vi "TF+NLH_2Dsweep.vi"() -> ()   [LabVIEW 2022 SP3]
uses:
  <vilib>/Analysis/baseanly.llb/Mean (DBL).vi
  <vilib>/Utility/file.llb/Write Delimited Spreadsheet (DBL).vi
  <vilib>/Analysis/NI_AALBase.lvlib
panel:
  in  "T Delay":dbl=3600.0
  out "Temperature":dbl
  out "Field":dbl
  out "Field Status 2":i32(ring) items=["MagnetUnknown"=0, "StablePersistent"=1, "WarmingSwitch"=2, "CoolingSwitch"=3, "StableDriven"=4, "Iterating"=5, "Charging"=6, "Discharging"=7, "CurrentError"=8, "MagnetFailure"=15]
  out "Temperature Status 2":i32(ring) items=["TemperatureUnknown"=0, "Stable"=1, "Tracking"=2, "Near"=5, "Chasing"=6, "Filling"=7, "Standby"=10, "Disabled"=13, "ImpedanceNotFunction"=14, "TempFailure"=15]
  in  "?":bool
  out "Sine voltage F":dbl format="%#_13g"
  out "Sine voltage T":dbl format="%#_13g"
  in  "Initialize after measurement":bool
  in  "F Delay":dbl=5.0
  out "PhaseA-F":cluster{dbl[], dbl[]}(graph)
  out "RA-F":cluster{dbl[], dbl[]}(graph)
  out "Phaseh1-F":cluster{dbl[], dbl[]}(graph)
  out "Rh1B-F":cluster{dbl[], dbl[]}(graph)
  out "phase B 2":dbl
  in  "Phase B 2":u16(ring)=9 items=["X", "Y", "R", "Theta", "Frequency", "Noise", "Xh1", "Yh1", "Rh1", "Theta h1", "Xh2", "Yh2", "Rh2", "Theta h2"]
  out "phase A 2":dbl
  in  "Phase A 2":u16(ring)=3 items=["X", "Y", "R", "Theta", "Frequency", "Noise", "Xh1", "Yh1", "Rh1", "Theta h1", "Xh2", "Yh2", "Rh2", "Theta h2"]
  out "para1 Measurement (mV) 2":dbl=1.49013e-07
  in  "F Clear Plot A":bool
  in  "Parameter A 2":u16(ring)=2 items=["X", "Y", "R", "Theta", "Frequency", "Noise", "Xh1", "Yh1", "Rh1", "Theta h1", "Xh2", "Yh2", "Rh2", "Theta h2"]
  out "para2 Measurement (uV) 2":dbl=1.49013e-07
  in  "F Clear Plot B":bool
  in  "Parameter B 2":u16(ring)=8 items=["X", "Y", "R", "Theta", "Frequency", "Noise", "Xh1", "Yh1", "Rh1", "Theta h1", "Xh2", "Yh2", "Rh2", "Theta h2"]
  out "V Loop Run F":i32
  out "Backward":bool
  out "Forward":bool
  in  "V Step(mV)":i32=20
  out "V Loop Run T":i32
  in  "V Loop#":i32=1
  in  "High Value (V)":dbl=3.0
  in  "Low Value (V)":dbl=0.1
  in  "Series Resistance":string="20kOhm"
  in  "System Stablization (s)":dbl=0.1 format="%#_13g"
  in  "Low Value (Oe)":dbl
  in  "High Value (Oe)":dbl=70000.0
  in  "Sweep Field Approach":i32(ring) items=["Linear", "NoOvershoot", "Oscillate"]
  in  "Sweep F Rate (Oe/s)":dbl=200.0 format="%#_13g"
  in  "Sweep F mode":i32(ring) items=["Persistent", "Driven"]
  in  "Set Fixed T":dbl=300.0
  in  "Fixed Temperature Approach":i32(ring)=1 items=["FastSettle", "NoOvershoot"]
  in  "FIxed T  Rate (K/min)":dbl=20.0
  out "Field Setting":dbl format="%#_13g"
  out "Fixed Temperature":dbl
  out "Measured Field":dbl
  out "Field Status":i32(ring) items=["MagnetUnknown"=0, "StablePersistent"=1, "WarmingSwitch"=2, "CoolingSwitch"=3, "StableDriven"=4, "Iterating"=5, "Charging"=6, "Discharging"=7, "CurrentError"=8, "MagnetFailure"=15]
  out "Temperature Status":i32(ring) items=["TemperatureUnknown"=0, "Stable"=1, "Tracking"=2, "Near"=5, "Chasing"=6, "Filling"=7, "Standby"=10, "Disabled"=13, "ImpedanceNotFunction"=14, "TempFailure"=15]
  out "Measuring F":bool
  in  "Step(Oe)":i32=5000
  out "Temperature Status":i32(ring) items=["TemperatureUnknown"=0, "Stable"=1, "Tracking"=2, "Near"=5, "Chasing"=6, "Filling"=7, "Standby"=10, "Disabled"=13, "ImpedanceNotFunction"=14, "TempFailure"=15]
  out "Field Status":i32(ring) items=["MagnetUnknown"=0, "StablePersistent"=1, "WarmingSwitch"=2, "CoolingSwitch"=3, "StableDriven"=4, "Iterating"=5, "Charging"=6, "Discharging"=7, "CurrentError"=8, "MagnetFailure"=15]
  out "Fixed Field":dbl
  out "Measured Temperature":dbl
  in  "Set FIxed F (Oe)":dbl format="%#_13g"
  in  "Fixed Field Approach":i32(ring) items=["Linear", "NoOvershoot", "Oscillate"]
  in  "FIxed F Rate (Oe/s)":dbl=100.0 format="%#_13g"
  in  "Fixed F mode":i32(ring) items=["Persistent", "Driven"]
  in  "Sweep Temperature Approach":i32(ring)=1 items=["FastSettle", "NoOvershoot"]
  in  "Sweep T  Rate (K/min)":dbl=10.0
  in  "Sweep T/F":bool=TRUE
  in  "Remote":bool=TRUE
  in  "IP Address":string="169.254.170.239"
  out "Measuring T":bool
  in  "path (folder + filename)":string="G:\\My Drive\\Opticool\\Measurement\\NLH\\T dependence\\TaI23_A67_B68_267Hz"
  in  "LOCKIN address":refnum<visa-resource-name>="COM3"
  out "PhaseA-T":cluster{dbl[], dbl[]}(graph)
  out "RA-T":cluster{dbl[], dbl[]}(graph)
  out "Phaseh1-T":cluster{dbl[], dbl[]}(graph)
  out "Rh1B-T":cluster{dbl[], dbl[]}(graph)
  out "phase B":dbl
  in  "Phase B":u16(ring)=9 items=["X", "Y", "R", "Theta", "Frequency", "Noise", "Xh1", "Yh1", "Rh1", "Theta h1", "Xh2", "Yh2", "Rh2", "Theta h2"]
  out "phase A":dbl
  in  "Phase A":u16(ring)=3 items=["X", "Y", "R", "Theta", "Frequency", "Noise", "Xh1", "Yh1", "Rh1", "Theta h1", "Xh2", "Yh2", "Rh2", "Theta h2"]
  out "para1 Measurement (mV)":dbl=1.49013e-07
  in  "T Clear Plot A":bool
  in  "Parameter A":u16(ring)=2 items=["X", "Y", "R", "Theta", "Frequency", "Noise", "Xh1", "Yh1", "Rh1", "Theta h1", "Xh2", "Yh2", "Rh2", "Theta h2"]
  out "para2 Measurement (uV)":dbl=1.49013e-07
  in  "T Clear Plot B":bool
  in  "Parameter B":u16(ring)=8 items=["X", "Y", "R", "Theta", "Frequency", "Noise", "Xh1", "Yh1", "Rh1", "Theta h1", "Xh2", "Yh2", "Rh2", "Theta h2"]
  out "Temperature Setting":dbl format="%#_13g"
  in  "Save data or not":bool=TRUE
  in  "Step(K)":i32=10
  in  "B frequency":dbl=267.77 format="%#_13g"
  in  "B Input Connection (0: Single-Ended)":u16(ring)=1 items=["Single-Ended Voltage", "Differential Voltage", "1 MOhm Current Gain", "100 MOhm Current Gain"]
  in  "B harmonic 1":u8=2
  in  "B harmonic 2":u8=3
  in  "B reference Manual Phase":dbl=90.0
  in  "auto phase B":bool=TRUE
  in  "B Sample time (s)":dbl=0.001 min=0.001 max=100.0 step=0.001
  in  "B Sensitivity":u16(ring)=21 items=["1 nV/fA", "2 nV/fA", "5 nV/fA", "10 nV/fA", "20 nV/fA", "50 nV/fA", "100 nV/fA", "200 nV/fA", "500 nV/fA", "1 uV/pA", "2 uV/pA", "5 uV/pA", "10 uV/pA", "20 uV/pA", "50 uV/pA", "100 uV/pA", "200 uV/pA", "500 uV/pA", "1 mV/nA", "2 mV/nA", "5 mV/nA", "10 mV/nA", "20 mV/nA", "50 mV/nA", "100 mV/nA", "200 mV/nA", "500 mV/nA", "1 V/uA"]
  in  "Enable Sync Filter B (open when f<200Hz)":bool
  in  "B Time Constant":u8(ring)=9 items=["10 us", "30 us", "100 us", "300 us", "1 ms", "3 ms", "10 ms", "30 ms", "100 ms", "300 ms", "1 s", "3 s", "10 s", "30 s", "100 s", "300 s", "1 ks", "3 ks"]
  in  "B Reference Source":u8(ring) items=["External", "Internal", "Internal Sweep", "Channel-A"]
  in  "B Low Pass Filter Slope":u8(ring)=2 items=["6 dB/oct", "12 dB/oct", "18 db/oct", "24 dB/oct"]
  in  "A frequency":dbl=267.77 format="%#_13g"
  in  "A Input Connection (0: Single-Ended)":u16(ring)=1 items=["Single-Ended Voltage", "Differential Voltage", "1 MOhm Current Gain", "100 MOhm Current Gain"]
  in  "A harmonic 1":u8=2
  in  "A harmonic 2":u8=3
  in  "A reference Manual Phase":dbl
  in  "auto phase A":bool=TRUE
  in  "A Reference Source":u8(ring)=1 items=["External", "Internal", "Internal Sweep"]
  in  "A Sample time (s)":dbl=0.001 min=0.001 max=100.0 step=0.001
  in  "A Time Constant":u8(ring)=8 items=["10 us", "30 us", "100 us", "300 us", "1 ms", "3 ms", "10 ms", "30 ms", "100 ms", "300 ms", "1 s", "3 s", "10 s", "30 s", "100 s", "300 s", "1 ks", "3 ks"]
  in  "Enable Sync Filter A (open when f<200Hz)":bool
  in  "A Sensitivity":u16(ring)=21 items=["1 nV/fA", "2 nV/fA", "5 nV/fA", "10 nV/fA", "20 nV/fA", "50 nV/fA", "100 nV/fA", "200 nV/fA", "500 nV/fA", "1 uV/pA", "2 uV/pA", "5 uV/pA", "10 uV/pA", "20 uV/pA", "50 uV/pA", "100 uV/pA", "200 uV/pA", "500 uV/pA", "1 mV/nA", "2 mV/nA", "5 mV/nA", "10 mV/nA", "20 mV/nA", "50 mV/nA", "100 mV/nA", "200 mV/nA", "500 mV/nA", "1 V/uA"]
  in  "A Low Pass Filter Slope":u8(ring)=2 items=["6 dB/oct", "12 dB/oct", "18 db/oct", "24 dB/oct"]
  in  "stabilization(S)":dbl=0.1 format="%#_13g"
  in  "End Value (K)":dbl=302.0
  in  "Start Value (K)":dbl=2.0
  in  "Single/Double":i32=2 min=1 max=2 step=1
  # "Statue"
  # "Lock-in Setting"
  # "Channel B"
  # "Channel A"
  # "Sweep Setting"
  # "Sweep F Mesurement"
  # "Temprature and Field Setting"
  # "Sweep T Mesurement"
  # "Sweep F"
  # "Sweep T"
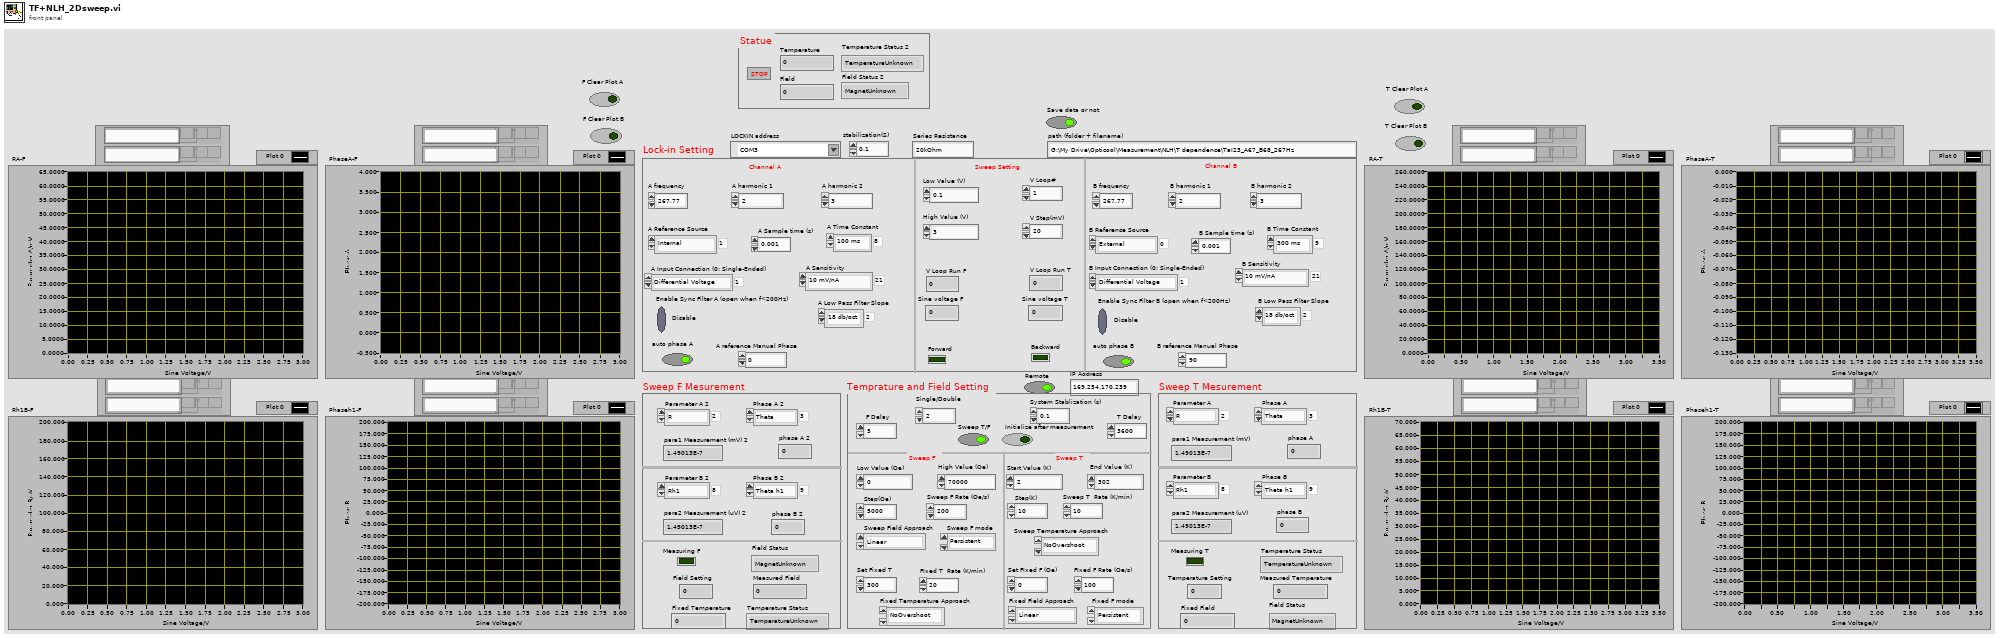
[diagram p1: front panel]
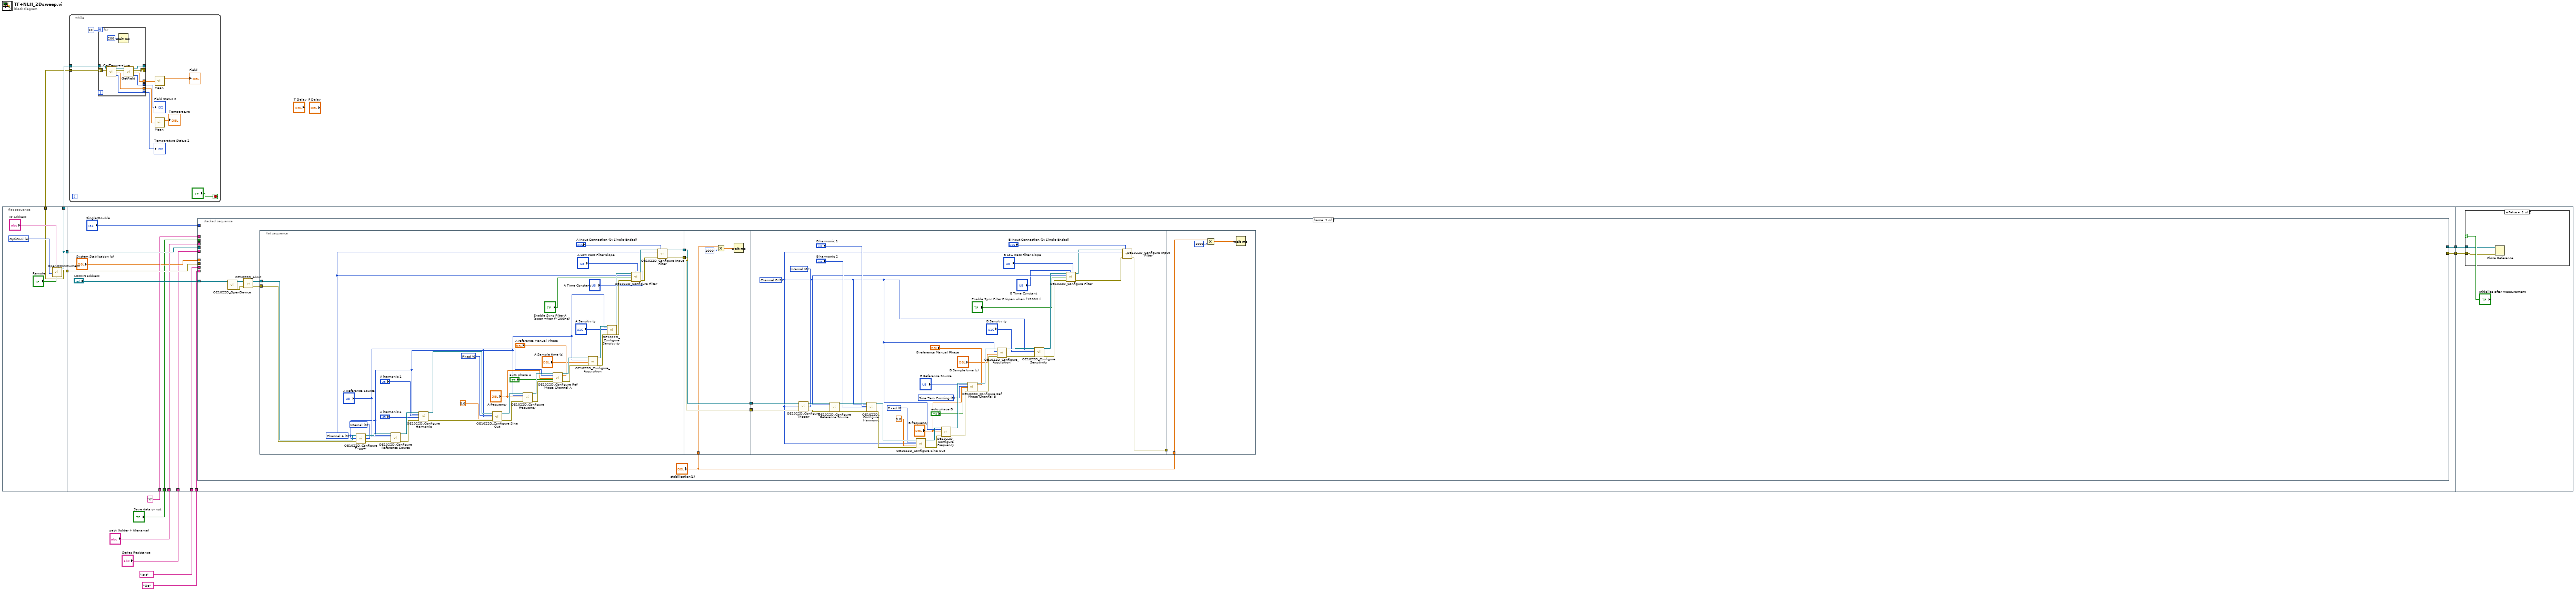
[diagram p0: block diagram]
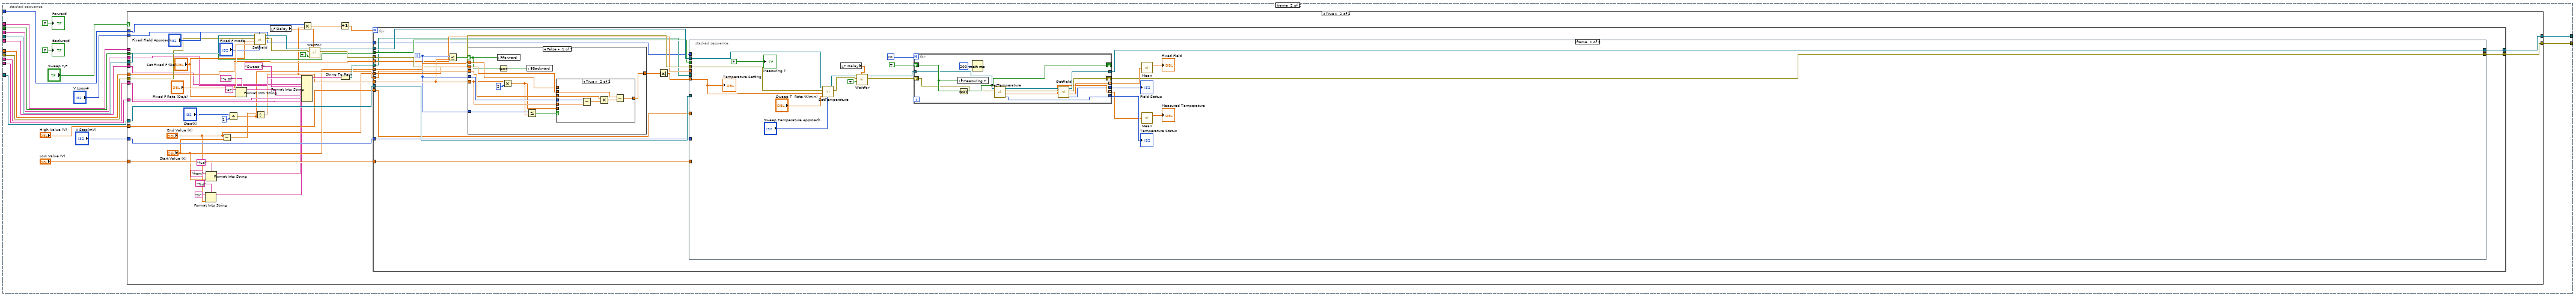
[diagram p2: hidden frame]
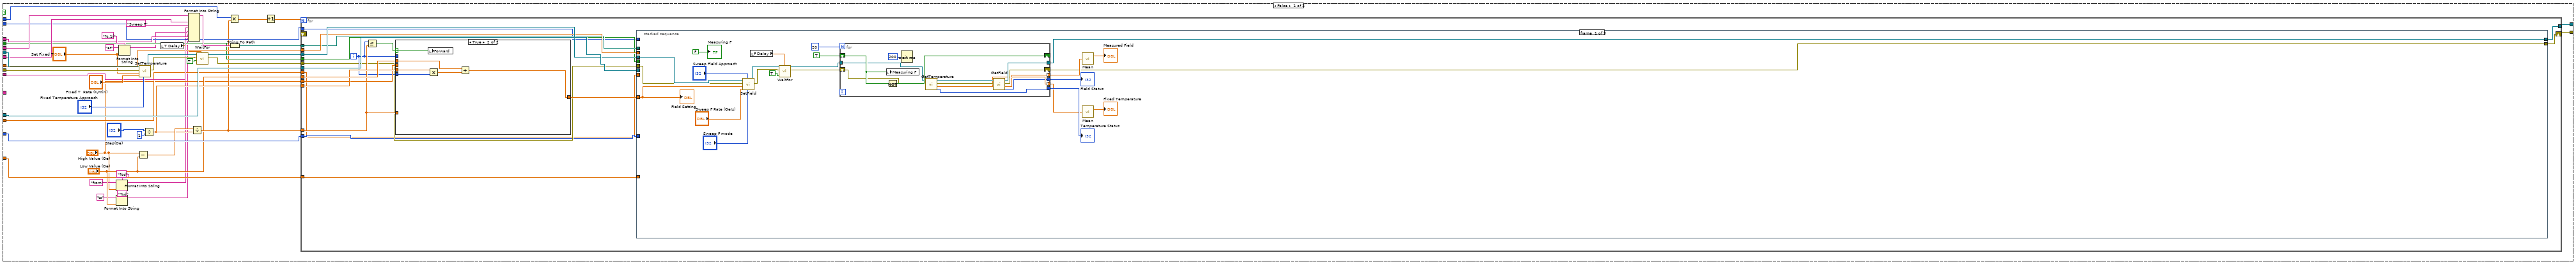
[diagram p3: hidden frame]
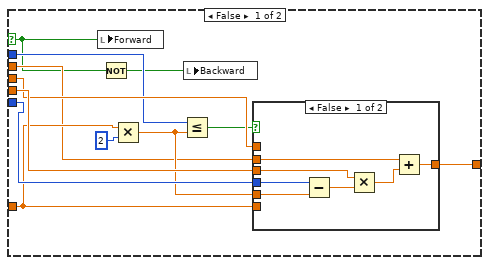
[diagram p4: hidden frame]
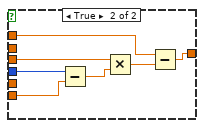
[diagram p5: hidden frame]
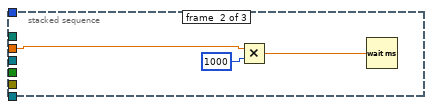
[diagram p6: hidden frame]
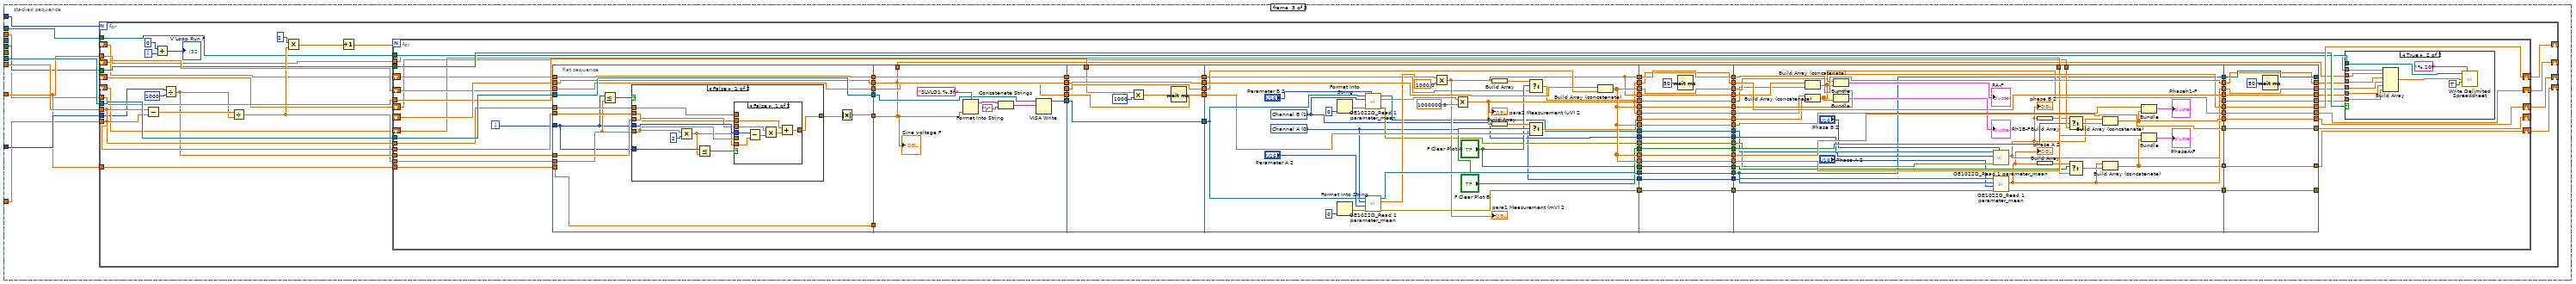
[diagram p7: hidden frame]
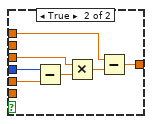
[diagram p9: hidden frame]
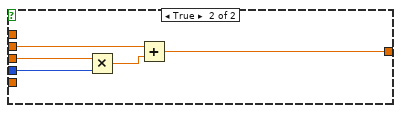
[diagram p10: hidden frame]
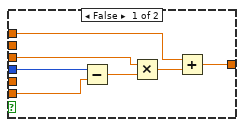
[diagram p11: hidden frame]
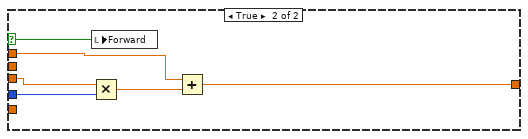
[diagram p12: hidden frame]
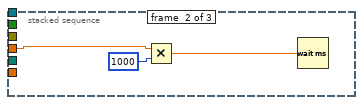
[diagram p13: hidden frame]
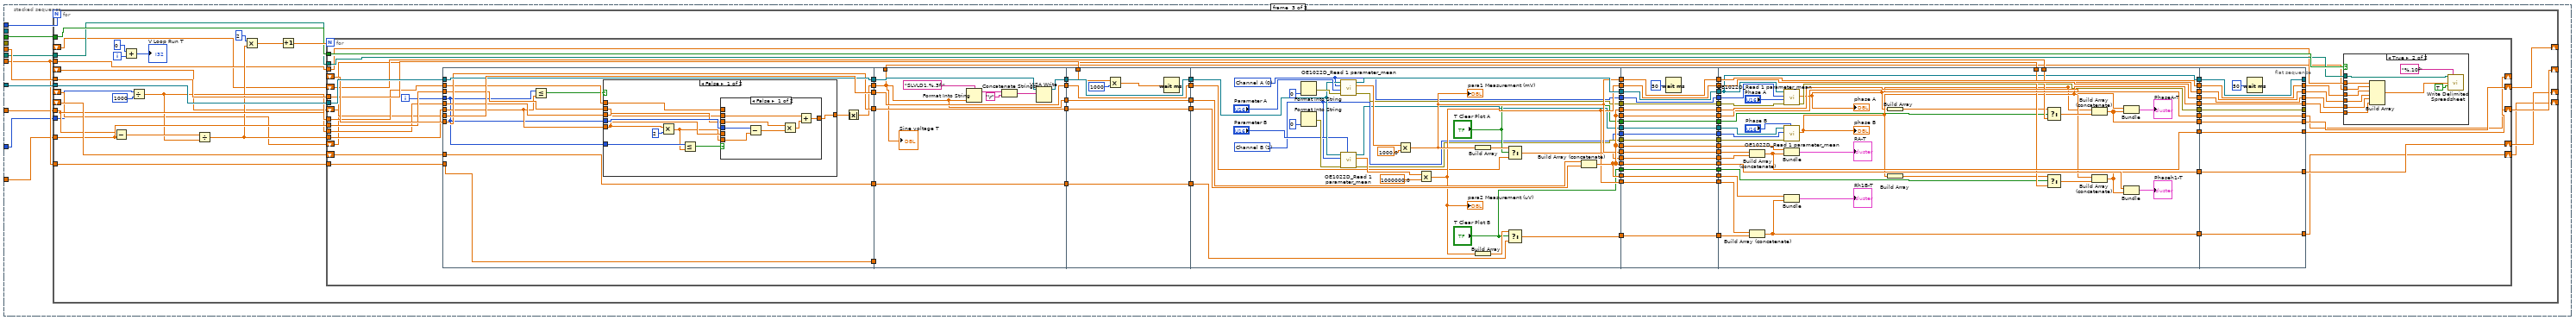
[diagram p14: hidden frame]
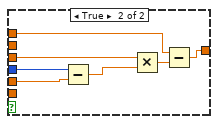
[diagram p16: hidden frame]
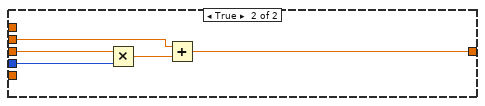
[diagram p17: hidden frame]
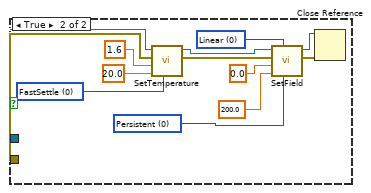
[diagram p18: hidden frame]
diagram:
  n1 = flat-sequence {
    tunnel: [w14] -> w12
    tunnel: [w13] -> w11
    tunnel: [w14] -> w2
    tunnel: [w13] -> w1
    tunnel: w12 -> [w28]
    tunnel: w11 -> [w27]
    tunnel: "path (folder + filename)" -> [w26]
    tunnel: "Oe" -> [w25]
    tunnel: "K" -> [w24]
    tunnel: ".txt" -> [w23]
    tunnel: [w21] -> w6
    tunnel: [w20] -> w5
    tunnel: "Series Resistance" -> [w19]
    tunnel: "Save data or not" -> [w18]
    tunnel: w6 -> [w1015]
    tunnel: w5 -> [w1014]
    frame #0 {
      w15 = 4 items=["PPMS", "VersaLab", "DynaCool", "SVSM", "OptiCool"] ("InstrumentType")
      n2 = call "OpenQDInstrument.vi"("Remote"="Remote", "IP Address"="IP Address", "InstrumentType"=w15) -> ("error out"=w13:errorcluster, "Instrument Ref"=w14:refnum<k24>)  [unwired: 5 in]
    }
    frame #1 {
      n3 = stacked-sequence {
        tunnel: "LOCKIN address" -> [w33 w145]
        tunnel: "Single/Double" -> [_ w144]
        tunnel: w28 -> [_ w142]
        tunnel: w27 -> [_ w141]
        tunnel: w26 -> [_ w140]
        tunnel: w25 -> [_ w139]
        tunnel: w24 -> [_ w138]
        tunnel: w23 -> [_ w137]
        tunnel: "System Stablization (s)" -> [_ w136]
        tunnel: [_ w135] -> w21
        tunnel: [_ w134] -> w20
        tunnel: w19 -> [_ w133]
        tunnel: w18 -> [_ w132]
        frame #0 {
          n4 = call <instrlib>:"OE1022D_OpenDevice.vi"("VISA resource name"=w33) -> ("VISA资源名称输出"=w32:refnum<visa-resource-name>, "错误输出"=w34:errorcluster)  [unwired: 17 in]
          n5 = call <instrlib>:"OE1022D_Abort.vi"("error in (no error)"=w34, "VISA resource name"=w32) -> ("error out"=w39:errorcluster, "VISA resource name out"=w40:refnum<visa-resource-name>)
          n6 = flat-sequence {
            tunnel: w40 -> [w79]
            tunnel: [w67] -> w38
            tunnel: w39 -> [w78]
            tunnel: [w55] -> w36
            tunnel: w38 -> [w84]
            tunnel: [w84] -> w37
            tunnel: w36 -> [w83]
            tunnel: [w83] -> w35
            tunnel: "stabilization(S)" -> [w80]
            tunnel: w37 -> [w105]
            tunnel: [w104] -> w41
            tunnel: w35 -> [w103]
            tunnel: w41 -> [_]
            tunnel: "stabilization(S)" -> [w123]
            frame #0 {
              w54 = u8 0 items=["Fixed", "Linear", "Log"] ("SineOut Mode")
              w56 = u16 0 items=["Internal", "External"] ("Trigger Source (0: Internal)")
              w45 = u8 0 items=["Channel A", "Channel B"] ("OE1022D A/B")
              n7 = call <instrlib>:"OE1022D_Configure Trigger.vi"("Trigger Source (0: Internal)"=w56, "error in (no error)   2"=w78, "OE1022D A/B"=w45, "VISA resource name   2"=w79) -> ("error out   2"=w72:errorcluster, "VISA resource name out   2"=w73:refnum<visa-resource-name>)
              n8 = call <instrlib>:"OE1022D_Configure Reference Source.vi"("VISA resource name"=w73, "OE1022D A/B"=w45, "Reference Source"="A Reference Source", "error in (no error)"=w72) -> ("VISA resource name out"=w71:refnum<visa-resource-name>, "error out"=w69:errorcluster)  [unwired: 14 in]
              n9 = call <instrlib>:"OE1022D_Configure Harmonic.vi"("VISA resource name"=w71, "OE1022D A/B"=w45, "Harmonic 1"="A harmonic 1", "Harmonic 2"="A harmonic 2", "error in (no error)"=w69) -> ("VISA resource name out"=w70:refnum<visa-resource-name>, "error out"=w68:errorcluster)  [unwired: 13 in]
              n10 = call <instrlib>:"OE1022D_Configure Sine Out.vi"("VISA resource name"=w70, "SineOut Mode"=w54, "OE1022D A/B"=w45, "Sine Output Amplitude (V)"=sgl 0.0 ("A Sine Output Amplitude (V)"), "error in (no error)"=w68) -> ("VISA resource name out"=w76:refnum<visa-resource-name>, "error out"=w75:errorcluster)  [unwired: 9 in]
              n11 = call <instrlib>:"OE1022D_Configure Frequency.vi"("VISA resource name"=w76, "OE1022D A/B"=w45, "Internal Frequency(Hz)"="A frequency", "error in (no error)"=w75) -> ("VISA resource name out"=w66:refnum<visa-resource-name>, "error out"=w63:errorcluster)  [unwired: 14 in]
              n12 = call <instrlib>:"OE1022D_Configure Ref Phase Channel A.vi"("VISA resource name"=w66, "Reference Source"="A Reference Source", "Internal Frequency(Hz)"="A frequency", "Auto Phase (T: Enabled)"="auto phase A", "error in (no error)"=w63, "Manual Phase  (degree)"="A reference Manual Phase") -> ("VISA resource name out"=w65:refnum<visa-resource-name>, "error out"=w64:errorcluster)  [unwired: 12 in]
              n13 = call <instrlib>:"OE1022D_Configure_Acquisition.vi"("VISA resource name"=w65, "OE1022D A/B"=w45, "Sample time (s)"="A Sample time (s)", "error in (no error)"=w64) -> ("VISA resource name out"=w48:refnum<visa-resource-name>, "error out"=w47:errorcluster)  [unwired: 4 in]
              n14 = call <instrlib>:"OE1022D_Configure Sensitivity.vi"("VISA resource name"=w48, "OE1022D A/B"=w45, "Sensitivity"="A Sensitivity", "error in (no error)"=w47) -> ("VISA resource name out"=w52:refnum<visa-resource-name>, "error out"=w51:errorcluster)  [unwired: 14 in]
              n15 = call <instrlib>:"OE1022D_Configure Filter.vi"("Low Pass Filter Slope (1: 12dB/oct)"="A Low Pass Filter Slope", "Time Constant (8: 100ms)"="A Time Constant", "error in (no error)"=w51, "Enable Sync Filter (F: Disable)"="Enable Sync Filter A (open when f<200Hz)", "OE1022D A/B"=w45, "VISA resource name"=w52) -> ("error out"=w49:errorcluster, "VISA resource name out"=w50:refnum<visa-resource-name>)  [unwired: 4 in]
              n16 = call <instrlib>:"OE1022D_Configure Input Filter.vi"("VISA resource name"=w50, "Input Source"="A Input Connection (0: Single-Ended)", "OE1022D A/B"=w45, "error in (no error)"=w49) -> ("VISA resource name out"=w55:refnum<visa-resource-name>, "error out"=w67:errorcluster)  [unwired: 10 in]
            }
            frame #1 {
              n17 = Multiply(x=w80, y=1000) -> (x*y=w82:dbl)
              n18 = Wait (ms)(milliseconds to wait=w82) -> ()  [unwired: 1 out]
            }
            frame #2 {
              w87 = u8 2 items=["TTL Pos", "TTL Neg", "Sine Zero Crossing"] ("External Ref Trigger")
              w100 = u8 0 items=["Fixed", "Linear", "Log"] ("SineOut Mode")
              w106 = u16 0 items=["Internal", "External"] ("Trigger Source (0: Internal)")
              w92 = u8 1 items=["Channel A", "Channel B"] ("OE1022D A/B")
              n19 = call <instrlib>:"OE1022D_Configure Trigger.vi"("Trigger Source (0: Internal)"=w106, "error in (no error)   2"=w105, "OE1022D A/B"=w92, "VISA resource name   2"=w103) -> ("error out   2"=w118:errorcluster, "VISA resource name out   2"=w119:refnum<visa-resource-name>)
              n20 = call <instrlib>:"OE1022D_Configure Reference Source.vi"("VISA resource name"=w119, "OE1022D A/B"=w92, "error in (no error)"=w118) -> ("VISA resource name out"=w117:refnum<visa-resource-name>, "error out"=w115:errorcluster)  [unwired: 15 in]
              n21 = call <instrlib>:"OE1022D_Configure Harmonic.vi"("VISA resource name"=w117, "OE1022D A/B"=w92, "Harmonic 1"="B harmonic 1", "Harmonic 2"="B harmonic 2", "error in (no error)"=w115) -> ("VISA resource name out"=w116:refnum<visa-resource-name>, "error out"=w114:errorcluster)  [unwired: 13 in]
              n22 = call <instrlib>:"OE1022D_Configure Sine Out.vi"("VISA resource name"=w116, "SineOut Mode"=w100, "OE1022D A/B"=w92, "Sine Output Amplitude (V)"=sgl 0.0, "error in (no error)"=w114) -> ("VISA resource name out"=w121:refnum<visa-resource-name>, "error out"=w120:errorcluster)  [unwired: 9 in]
              n23 = call <instrlib>:"OE1022D_Configure Frequency.vi"("VISA resource name"=w121, "OE1022D A/B"=w92, "Internal Frequency(Hz)"="B frequency", "error in (no error)"=w120) -> ("VISA resource name out"=w113:refnum<visa-resource-name>, "error out"=w110:errorcluster)  [unwired: 14 in]
              n24 = call <instrlib>:"OE1022D_Configure Ref Phase Channel B.vi"("VISA resource name"=w113, "Reference Source"="B Reference Source", "External Ref Trigger"=w87, "Internal Frequency(Hz)"="B frequency", "Auto Phase (T: Enabled)"="auto phase B", "error in (no error)"=w110, "Manual Phase  (degree)"="B reference Manual Phase") -> ("VISA resource name out"=w112:refnum<visa-resource-name>, "error out"=w111:errorcluster)  [unwired: 11 in]
              n25 = call <instrlib>:"OE1022D_Configure_Acquisition.vi"("VISA resource name"=w112, "OE1022D A/B"=w92, "Sample time (s)"="B Sample time (s)", "error in (no error)"=w111) -> ("VISA resource name out"=w93:refnum<visa-resource-name>, "error out"=w94:errorcluster)  [unwired: 4 in]
              n26 = call <instrlib>:"OE1022D_Configure Sensitivity.vi"("VISA resource name"=w93, "OE1022D A/B"=w92, "Sensitivity"="B Sensitivity", "error in (no error)"=w94) -> ("VISA resource name out"=w97:refnum<visa-resource-name>, "error out"=w96:errorcluster)  [unwired: 14 in]
              n27 = call <instrlib>:"OE1022D_Configure Filter.vi"("Low Pass Filter Slope (1: 12dB/oct)"="B Low Pass Filter Slope", "Time Constant (8: 100ms)"="B Time Constant", "error in (no error)"=w96, "Enable Sync Filter (F: Disable)"="Enable Sync Filter B (open when f<200Hz)", "OE1022D A/B"=w92, "VISA resource name"=w97) -> ("error out"=w95:errorcluster, "VISA resource name out"=w85:refnum<visa-resource-name>)  [unwired: 4 in]
              n28 = call <instrlib>:"OE1022D_Configure Input Filter.vi"("VISA resource name"=w85, "Input Source"="B Input Connection (0: Single-Ended)", "OE1022D A/B"=w92, "error in (no error)"=w95) -> ("error out"=w104:errorcluster)  [unwired: 10 in, 1 out]
            }
            frame #3 {
              n29 = Multiply(x=w123, y=1000) -> (x*y=w125:dbl)
              n30 = Wait (ms)(milliseconds to wait=w125) -> ()  [unwired: 1 out]
            }
          }
        }
        frame #1 {
          n31 = case shown="True" "Sweep T/F" {
            tunnel: w145 -> [w191 w625]
            tunnel: w144 -> [w157 w624]
            tunnel: w142 -> [w184 w620]
            tunnel: w141 -> [w185 w619]
            tunnel: w140 -> [w177 w609]
            tunnel: w139 -> [_ w601]
            tunnel: w138 -> [w170 _]
            tunnel: w137 -> [w176 w607]
            tunnel: w136 -> [w175 w606]
            tunnel: [w174 w605] -> w135
            tunnel: [w173 w604] -> w134
            tunnel: w133 -> [w172 w603]
            tunnel: w132 -> [w166 w600]
            tunnel: "V Step(mV)" -> [w169 w592]
            tunnel: "High Value (V)" -> [w167 w591]
            tunnel: "Low Value (V)" -> [w168 w590]
            tunnel: "V Loop#" -> [w165 w589]
            frame False {
              n32 = Format Into String(format string="%d", initial string="from", "High Value (Oe)") -> (resulting string=w148:string)  [unwired: 1 in, 1 out]
              n33 = Format Into String(format string="%d", initial string="to", "Low Value (Oe)") -> (resulting string=w147:string)  [unwired: 1 in, 1 out]
              n34 = Format Into String(format string="%.1f", initial string="at", "Set Fixed T") -> (resulting string=w156:string)  [unwired: 1 in, 1 out]
              n35 = Subtract(x="High Value (Oe)", y="Low Value (Oe)") -> (x-y=w162:dbl)
              n36 = call "SetTemperature.vi"("Approach"="Fixed Temperature Approach", "Rate"="FIxed T  Rate (K/min)", "Temperature"="Set Fixed T", "error in (no error)"=w185, "Instrument Ref In"=w184) -> ("error out"=w186:errorcluster, "Instrument Ref Out"=w187:refnum<k24>)  [unwired: 2 in, 1 out]
              n37 = Divide(x="Step(Oe)", y=1) -> (x/y=w161:dbl)
              n38 = local read "T Delay"() -> (w146:dbl)
              n39 = Format Into String(initial string=w177, w172, "Sweep F", w148, w147, w156, w170, w176) -> (resulting string=w179:string)  [unwired: 2 in, 1 out]
              n40 = Divide(x=w162, y=w161) -> (x/y=w160:dbl)
              n41 = call "WaitFor.vi"("Delay"=w146, "Wait For Temperature"=TRUE ("WaitForTemperature"), "error in (no error)"=w186, "Instrument Ref In"=w187) -> ("error out"=w183:errorcluster, "Instrument Ref Out"=w182:refnum<k24>)  [unwired: 6 in]
              n42 = Multiply(x=w157, y=w160) -> (x*y=w159:dbl)
              n43 = String To Path(string=w179) -> (path=w178:path)
              n44 = Increment(x=w159) -> (x+1=w158:dbl)
              n45 = for {
                N: w158 -> [_]
                tunnel: w191 -> [w210]
                tunnel: w161 -> [w207]
                tunnel: w160 -> [w205]
                tunnel: "Low Value (Oe)" -> [w208]
                tunnel: "High Value (Oe)" -> [w206]
                tunnel: w178 -> [w197]
                tunnel: w182 -> [w202]
                tunnel: w183 -> [w201]
                tunnel: w175 -> [w200]
                shift-right: [w199] -> w174
                shift-left: _ -> [_]
                tunnel: [w198] -> w173
                tunnel: w169 -> [w196]
                tunnel: w168 -> [w195]
                tunnel: w167 -> [w194]
                tunnel: w166 -> [w193]
                tunnel: w165 -> [w192]
                i -> [w204]
                n46 = Less Or Equal?(x=w204, y=w205) -> (x <= y?=w209:bool)
                n47 = case shown="True" w209 {
                  selector: w209 -> [w211 w237]
                  tunnel: w208 -> [w213 w242]
                  tunnel: w204 -> [w222 w241]
                  tunnel: w207 -> [w221 w240]
                  tunnel: [w219 w238] -> w203
                  tunnel: w206 -> [w220 _]
                  tunnel: w205 -> [w215 _]
                  tunnel: w204 -> [w218 _]
                  frame False {
                    n48 = local write "Forward"(w211) -> ()
                    n49 = Not(x=w211) -> (.not. x?=w212:bool)
                    n50 = Multiply(x=w215, y=2) -> (x*y=w214:dbl)
                    n51 = Less Or Equal?(x=w218, y=w214) -> (x <= y?=w216:bool)
                    n52 = local write "Backward"(w212) -> ()
                    n53 = case shown="False" w216 {
                      tunnel: w222 -> [w229 w236]
                      tunnel: w221 -> [w227 w234]
                      tunnel: w220 -> [_ w232]
                      tunnel: [w225 w231] -> w219
                      tunnel: w215 -> [_ w230]
                      tunnel: w214 -> [w224 _]
                      tunnel: w213 -> [w223 _]
                      frame False {
                        n54 = Subtract(x=w229, y=w224) -> (x-y=w228:dbl)
                        n55 = Multiply(x=w227, y=w228) -> (x*y=w226:dbl)
                        n56 = Add(x=w223, y=w226) -> (x+y=w225:dbl)
                      }
                      frame True {
                        n57 = Subtract(x=w236, y=w230) -> (x-y=w235:dbl)
                        n58 = Multiply(x=w234, y=w235) -> (x*y=w233:dbl)
                        n59 = Subtract(x=w232, y=w233) -> (x-y=w231:dbl)
                      }
                    }
                  }
                  frame True {
                    n60 = Multiply(x=w240, y=w241) -> (x*y=w239:dbl)
                    n61 = local write "Forward"(w237) -> ()
                    n62 = Add(x=w242, y=w239) -> (x+y=w238:dbl)
                  }
                }
                n63 = stacked-sequence {
                  tunnel: w210 -> [_ _ w286]
                  tunnel: w203 -> [w248 _ w285]
                  tunnel: w202 -> [w247 _ _]
                  tunnel: w201 -> [w246 _ _]
                  tunnel: w200 -> [_ w279 w283]
                  tunnel: [w245 _ _] -> w199
                  tunnel: [w244 _ _] -> w198
                  tunnel: w197 -> [_ _ w290]
                  tunnel: w196 -> [_ _ w289]
                  tunnel: w195 -> [_ _ w288]
                  tunnel: w194 -> [_ _ w287]
                  tunnel: w193 -> [_ _ w284]
                  tunnel: w192 -> [_ _ w282]
                  frame #0 {
                    n64 = call "SetField.vi"("Mode"="Sweep F mode", "Approach"="Sweep Field Approach", "Rate"="Sweep F Rate (Oe/s)", "Field"=w248, "error in (no error)"=w246, "Instrument Ref In"=w247) -> ("error out"=w252:errorcluster, "Instrument Ref Out"=w253:refnum<k24>)  [unwired: 1 in, 1 out]
                    n65 = local read "F Delay"() -> (w243:dbl)
                    n66 = call "WaitFor.vi"("Delay"=w243, "Wait For Field"=TRUE, "error in (no error)"=w252, "Instrument Ref In"=w253) -> ("error out"=w250:errorcluster, "Instrument Ref Out"=w249:refnum<k24>)  [unwired: 6 in]
                    n67 = for {
                      N: 20 -> [_]
                      shift-right: [w278] -> _
                      shift-left: TRUE -> [w276]
                      shift-right: [w273] -> w245
                      shift-left: w250 -> [w275]
                      tunnel: w249 -> [w272]
                      tunnel: [w270] -> w244
                      tunnel: [w267] -> w263
                      tunnel: [w266] -> w262
                      tunnel: [w268] -> w260 mode=indexing
                      tunnel: [w269] -> w261 mode=indexing
                      n68 = local write "Measuring F"(w276) -> ()
                      n69 = Not(x=w276) -> (.not. x?=w278:bool)
                      n70 = Wait (ms)(milliseconds to wait=u32 200) -> ()  [unwired: 1 out]
                      n71 = call "GetTemperature.vi"("error in (no error)"=w275, "Instrument Ref In"=w272) -> ("Temperature\nStatus"=w266:i32, "Temperature"=w269:dbl, "error out"=w274:errorcluster, "Instrument Ref Out"=w271:refnum<k24>)  [unwired: 3 in, 1 out]
                      n72 = call "GetField.vi"("error in (no error)"=w274, "Instrument Ref In"=w271) -> ("Field\nStatus"=w267:i32, "Field"=w268:dbl, "error out"=w273:errorcluster, "Instrument Ref Out"=w270:refnum<k24>)  [unwired: 3 in, 1 out]
                    }
                    "Field Status" <- w263
                    "Temperature Status" <- w262
                    n73 = call-poly <vilib>:"Mean.vi"("X"=w260) -> ("mean"=→"Measured Field":dbl)  [unwired: 1 out]
                    n74 = call-poly <vilib>:"Mean.vi"("X"=w261) -> ("mean"=→"Fixed Temperature":dbl)  [unwired: 1 out]
                    "Field Setting" <- w248
                    "Measuring F" <- FALSE
                  }
                  frame #1 {
                    n75 = Multiply(x=w279, y=1000) -> (x*y=w281:dbl)
                    n76 = Wait (ms)(milliseconds to wait=w281) -> ()  [unwired: 1 out]
                  }
                  frame #2 {
                    n77 = for {
                      N: w282 -> [_]
                      tunnel: w286 -> [w316]
                      tunnel: w285 -> [w312]
                      tunnel: w283 -> [w308]
                      tunnel: w288 -> [w303]
                      tunnel: w287 -> [w301]
                      tunnel: w284 -> [w298]
                      tunnel: w290 -> [w297]
                      tunnel: w285 -> [w296]
                      shift-right: [w315] -> _
                      shift-left: _ -> [w295]
                      shift-right: [w317] -> _
                      shift-left: _ -> [w294]
                      shift-right: [w314] -> _
                      shift-left: _ -> [w293]
                      shift-right: [w292] -> _
                      shift-left: _ -> [w313]
                      tunnel: w289 -> [w291]
                      i -> [w311]
                      n78 = Subtract(x=w301, y=w303) -> (x-y=w305:dbl)
                      n79 = Add(x=0, y=w311) -> (x+y=→"V Loop Run F":i32)
                      n80 = Divide(x=w291, y=1000) -> (x/y=w300:dbl)
                      n81 = Divide(x=w305, y=w300) -> (x/y=w299:dbl)
                      n82 = Multiply(x=2, y=w299) -> (x*y=w304:dbl)
                      n83 = Increment(x=w304) -> (x+1=w302:dbl)
                      n84 = for {
                        N: w302 -> [_]
                        tunnel: w316 -> [w353]
                        tunnel: w312 -> [w348]
                        tunnel: w308 -> [w336]
                        tunnel: w303 -> [w335]
                        tunnel: w301 -> [w334]
                        tunnel: w300 -> [w333]
                        tunnel: w299 -> [w332]
                        tunnel: w298 -> [w330]
                        tunnel: w297 -> [w329]
                        tunnel: w296 -> [w328]
                        shift-right: [w351] -> w315
                        shift-left: w295 -> [w323]
                        shift-right: [w354] -> w317
                        shift-left: w294 -> [w322]
                        shift-right: [w350] -> w314
                        shift-left: w293 -> [w321]
                        shift-right: [w320] -> _
                        shift-left: _ -> [w352]
                        shift-right: [w319] -> w292
                        shift-left: w313 -> [w349]
                        i -> [w331]
                        n85 = flat-sequence {
                          tunnel: w349 -> [w427]
                          tunnel: w352 -> [w428]
                          tunnel: w348 -> [w429]
                          tunnel: w353 -> [w430]
                          tunnel: w322 -> [w431]
                          tunnel: [w431] -> w347
                          tunnel: [w430] -> w345
                          tunnel: [w429] -> w343
                          tunnel: [w428] -> w341
                          tunnel: [w427] -> w339
                          tunnel: [w419] -> w337
                          tunnel: w335 -> [w426]
                          tunnel: w334 -> [w425]
                          tunnel: w333 -> [w424]
                          tunnel: w332 -> [w423]
                          tunnel: w331 -> [w421]
                          tunnel: w347 -> [w470]
                          tunnel: [w470] -> w346
                          tunnel: w345 -> [w463]
                          tunnel: [w462] -> w344
                          tunnel: w343 -> [_]
                          tunnel: [w461] -> w342
                          tunnel: w341 -> [w469]
                          tunnel: [w469] -> w340
                          tunnel: w339 -> [w468]
                          tunnel: [w468] -> w338
                          tunnel: w337 -> [w461]
                          tunnel: [w461] -> w318
                          tunnel: w346 -> [w478]
                          tunnel: [w478] -> w408
                          tunnel: w344 -> [w477]
                          tunnel: [w477] -> w407
                          tunnel: w342 -> [w476]
                          tunnel: [w476] -> w406
                          tunnel: w340 -> [w475]
                          tunnel: [w475] -> w405
                          tunnel: w338 -> [w474]
                          tunnel: [w474] -> w404
                          tunnel: w336 -> [w471]
                          tunnel: [w503] -> w403
                          tunnel: [w490] -> w402
                          tunnel: [w491] -> w401
                          tunnel: [w488] -> w400
                          tunnel: [w491] -> w399
                          tunnel: [w491] -> w398
                          tunnel: [w491] -> w397
                          tunnel: [w491] -> w396
                          tunnel: [w490] -> w395
                          tunnel: [w489] -> w394
                          tunnel: [w488] -> w393
                          tunnel: [w487] -> w392
                          tunnel: ["F Clear Plot B"] -> w391
                          tunnel: ["F Clear Plot A"] -> w390
                          tunnel: [w484] -> w389
                          tunnel: [w483] -> w388
                          tunnel: [w482] -> w387
                          tunnel: [w481] -> w386
                          tunnel: [w480] -> w385
                          tunnel: w408 -> [w479]
                          tunnel: w407 -> [w498]
                          tunnel: w406 -> [w506]
                          tunnel: w405 -> [w505]
                          tunnel: w404 -> [w496]
                          tunnel: w403 -> [w528]
                          tunnel: [w528] -> w384
                          tunnel: w402 -> [w527]
                          tunnel: [w527] -> w383
                          tunnel: w401 -> [w526]
                          tunnel: [w526] -> w382
                          tunnel: w400 -> [w525]
                          tunnel: [w525] -> w381
                          tunnel: w399 -> [w524]
                          tunnel: [w524] -> w380
                          tunnel: w398 -> [w523]
                          tunnel: [w523] -> w379
                          tunnel: w397 -> [w522]
                          tunnel: [w522] -> w378
                          tunnel: w396 -> [w521]
                          tunnel: [w521] -> w377
                          tunnel: w395 -> [w520]
                          tunnel: [w520] -> w376
                          tunnel: w394 -> [w519]
                          tunnel: [w519] -> w375
                          tunnel: w393 -> [w518]
                          tunnel: [w518] -> w374
                          tunnel: w392 -> [w517]
                          tunnel: [w517] -> w373
                          tunnel: w391 -> [w516]
                          tunnel: [w516] -> w372
                          tunnel: w390 -> [w515]
                          tunnel: [w515] -> w371
                          tunnel: w389 -> [w514]
                          tunnel: [w514] -> w370
                          tunnel: w388 -> [w513]
                          tunnel: [w513] -> w369
                          tunnel: w387 -> [w512]
                          tunnel: [w512] -> w368
                          tunnel: w386 -> [w511]
                          tunnel: [w511] -> w367
                          tunnel: w385 -> [w510]
                          tunnel: [w510] -> w366
                          tunnel: w384 -> [w532]
                          tunnel: w383 -> [w566]
                          tunnel: w382 -> [w565]
                          tunnel: w381 -> [w564]
                          tunnel: w380 -> [w563]
                          tunnel: w379 -> [w561]
                          tunnel: w378 -> [w559]
                          tunnel: w377 -> [w557]
                          tunnel: w376 -> [w554]
                          tunnel: w375 -> [w553]
                          tunnel: w374 -> [w550]
                          tunnel: w373 -> [w549]
                          tunnel: w321 -> [w547]
                          tunnel: w372 -> [w546]
                          tunnel: w323 -> [w544]
                          tunnel: w371 -> [w543]
                          tunnel: w370 -> [w539]
                          tunnel: w369 -> [w538]
                          tunnel: w368 -> [w537]
                          tunnel: w367 -> [w534]
                          tunnel: w366 -> [w533]
                          tunnel: [w532] -> w365
                          tunnel: [w552] -> w364
                          tunnel: [w566] -> w363
                          tunnel: [w565] -> w362
                          tunnel: [w530] -> w361
                          tunnel: [w531] -> w360
                          tunnel: [w555] -> w359
                          tunnel: [w551] -> w358
                          tunnel: [w548] -> w357
                          tunnel: [w564] -> w356
                          tunnel: [w536] -> w355
                          tunnel: [w570] -> w324
                          tunnel: [w571] -> w327
                          tunnel: [w568] -> w319
                          tunnel: [w572] -> w350
                          tunnel: [w573] -> w351
                          tunnel: [w574] -> _
                          tunnel: [w575] -> w325
                          tunnel: [w576] -> w320
                          tunnel: [w577] -> w326
                          tunnel: [w567] -> w354
                          tunnel: [w578] -> _
                          tunnel: w365 -> [w578]
                          tunnel: w364 -> [w567]
                          tunnel: w363 -> [w577]
                          tunnel: w362 -> [w576]
                          tunnel: w361 -> [w575]
                          tunnel: w360 -> [w574]
                          tunnel: w359 -> [w573]
                          tunnel: w358 -> [w572]
                          tunnel: w357 -> [w568]
                          tunnel: w356 -> [w571]
                          tunnel: w355 -> [w570]
                          frame #0 {
                            n86 = Less Or Equal?(x=w421, y=w423) -> (x <= y?=w422:bool)
                            n87 = case shown="False" w422 {
                              tunnel: w426 -> [w432 w460]
                              tunnel: w421 -> [w441 w459]
                              tunnel: w424 -> [w440 w458]
                              tunnel: [w438 w456] -> w420
                              tunnel: w425 -> [w439 _]
                              tunnel: w423 -> [w434 _]
                              tunnel: w421 -> [w437 _]
                              frame False {
                                n88 = Multiply(x=w434, y=2) -> (x*y=w433:dbl)
                                n89 = Less Or Equal?(x=w437, y=w433) -> (x <= y?=w435:bool)
                                n90 = case shown="False" w435 {
                                tunnel: w441 -> [w448 w455]
                                tunnel: w440 -> [w446 w453]
                                tunnel: w439 -> [_ w451]
                                tunnel: [w444 w450] -> w438
                                tunnel: w434 -> [_ w449]
                                tunnel: w433 -> [w443 _]
                                tunnel: w432 -> [w442 _]
                                frame False {
                                n91 = Subtract(x=w448, y=w443) -> (x-y=w447:dbl)
                                n92 = Multiply(x=w446, y=w447) -> (x*y=w445:dbl)
                                n93 = Add(x=w442, y=w445) -> (x+y=w444:dbl)
                                }
                                frame True {
                                n94 = Subtract(x=w455, y=w449) -> (x-y=w454:dbl)
                                n95 = Multiply(x=w453, y=w454) -> (x*y=w452:dbl)
                                n96 = Subtract(x=w451, y=w452) -> (x-y=w450:dbl)
                                }
                                }
                              }
                              frame True {
                                n97 = Multiply(x=w458, y=w459) -> (x*y=w457:dbl)
                                n98 = Add(x=w460, y=w457) -> (x+y=w456:dbl)
                              }
                            }
                            n99 = Absolute Value(x=w420) -> (abs(x)=w419:dbl)
                          }
                          frame #1 {
                            n100 = Format Into String(format string="SLVLD1,%.3f;", w461) -> (resulting string=w465:string)  [unwired: 2 in, 1 out]
                            n101 = Concatenate Strings(w465, "\r") -> (w464:string)
                            n102 = VISA Write(VISA resource name=w463, write buffer=w464) -> (VISA resource name out=w462:refnum<visa-resource-name>)  [unwired: 1 in, 2 out]
                            "Sine voltage F" <- w461
                          }
                          frame #2 {
                            n103 = Multiply(x=w471, y=1000) -> (x*y=w473:dbl)
                            n104 = Wait (ms)(milliseconds to wait=w473) -> ()  [unwired: 1 out]
                          }
                          frame #3 {
                            w483 = u8 1 items=["Channel A", "Channel B"] ("Channel A/B for Parameter1")
                            w480 = u8 0 items=["Channel A", "Channel B"] ("Channel A/B for Parameter1")
                            n105 = Format Into String(0) -> (error out=w499:errorcluster)  [unwired: 3 in, 1 out]
                            n106 = Format Into String(0) -> (error out=w504:errorcluster)  [unwired: 3 in, 1 out]
                            n107 = call <instrlib>:"OE1022D_Read 1 parameter_mean.vi"("Parameter 2"="Parameter B 2", "错误输入（无错误）"=w499, "Channel (0: A)"=w483, "VISA resource name"=w498) -> ("error out"=w484:errorcluster, "Measurement"=w492:dbl, "VISA resource name out"=w482:refnum<visa-resource-name>)  [unwired: 5 in]
                            n108 = call <instrlib>:"OE1022D_Read 1 parameter_mean.vi"("错误输入（无错误）"=w504, "Parameter"="Parameter A 2", "Channel (0: A)"=w480, "VISA resource name"=w498) -> ("error out"=w481:errorcluster, "Measurement"=w493:dbl, "VISA resource name out"=w503:refnum<visa-resource-name>)  [unwired: 5 in]
                            n109 = Multiply(x=w493, y=1000.0) -> (x*y=w490:dbl)
                            "para1 Measurement (mV) 2" <- w490
                            n110 = Multiply(x=w492, y=1000000.0) -> (x*y=w488:dbl)
                            "para2 Measurement (uV) 2" <- w488
                            n111 = Build Array(w490) -> (w507:dbl[])
                            n112 = Build Array(w488) -> (w500:dbl[])
                            n113 = Select(t=w507, s="F Clear Plot A", f=w479) -> (s? t:f=w489:dbl[])
                            n114 = Select(t=w500, s="F Clear Plot B", f=w496) -> (s? t:f=w487:dbl[])
                            n115 = Build Array (concatenate)(w506, w505) -> (w491:dbl[])
                          }
                          frame #4 {
                            n116 = Wait (ms)(milliseconds to wait=u32 50) -> ()  [unwired: 1 out]
                          }
                          frame #5 {
                            n117 = Build Array (concatenate)(w554, w553) -> (w552:dbl[])
                            n118 = Build Array (concatenate)(w550, w549) -> (w548:dbl[])
                            n119 = Bundle(w559, w552) -> (→"RA-F":cluster{dbl[], dbl[]})  [unwired: 1 in]
                            n120 = Bundle(w561, w548) -> (→"Rh1B-F":cluster{dbl[], dbl[]})  [unwired: 1 in]
                            n121 = call <instrlib>:"OE1022D_Read 1 parameter_mean.vi"("Parameter 2"="Phase B 2", "错误输入（无错误）"=w539, "Channel (0: A)"=w538, "VISA resource name"=w537) -> ("Measurement"=w536:dbl)  [unwired: 5 in, 2 out]
                            "phase B 2" <- w536
                            n122 = call <instrlib>:"OE1022D_Read 1 parameter_mean.vi"("错误输入（无错误）"=w534, "Parameter"="Phase A 2", "Channel (0: A)"=w533, "VISA resource name"=w532) -> ("error out"=w531:errorcluster, "Measurement"=w530:dbl)  [unwired: 5 in, 1 out]
                            "phase A 2" <- w530
                            n123 = Build Array(w536) -> (w541:dbl[])
                            n124 = Build Array(w530) -> (w540:dbl[])
                            n125 = Select(t=w541, s=w546, f=w547) -> (s? t:f=w545:dbl[])
                            n126 = Select(t=w540, s=w543, f=w544) -> (s? t:f=w542:dbl[])
                            n127 = Build Array (concatenate)(w536, w545) -> (w551:dbl[])
                            n128 = Build Array (concatenate)(w530, w542) -> (w555:dbl[])
                            n129 = Bundle(w563, w551) -> (→"Phaseh1-F":cluster{dbl[], dbl[]})  [unwired: 1 in]
                            n130 = Bundle(w557, w555) -> (→"PhaseA-F":cluster{dbl[], dbl[]})  [unwired: 1 in]
                          }
                          frame #6 {
                            n131 = Wait (ms)(milliseconds to wait=u32 50) -> ()  [unwired: 1 out]
                          }
                        }
                        n132 = case shown="True" w330 {
                          tunnel: w329 -> [_ w417]
                          tunnel: w328 -> [_ w414]
                          tunnel: w327 -> [_ w412]
                          tunnel: w326 -> [_ w413]
                          tunnel: w325 -> [_ w411]
                          tunnel: w324 -> [_ w410]
                          tunnel: w318 -> [_ w409]
                          frame False {
                          }
                          frame True {
                            n133 = Build Array(w414, w409, w413, w411, w412, w410) -> (w416:dbl[])
                            n134 = call-poly <vilib>:"Write Delimited Spreadsheet.vi"("file path (dialog if empty)"=w417, "format (%.3f)"="%.10f", "1D data"=w416, "append to file? (new file:F)"=TRUE) -> ()  [unwired: 10 in, 2 out]
                          }
                        }
                      }
                    }
                  }
                }
              }
            }
            frame True {
              n135 = Format Into String(format string="%d", initial string="to", "End Value (K)") -> (resulting string=w580:string)  [unwired: 1 in, 1 out]
              n136 = Format Into String(format string="%d", initial string="from", "Start Value (K)") -> (resulting string=w581:string)  [unwired: 1 in, 1 out]
              n137 = Subtract(x="End Value (K)", y="Start Value (K)") -> (x-y=w597:dbl)
              n138 = Divide(x="Step(K)", y=1) -> (x/y=w596:dbl)
              n139 = Format Into String(format string="%.0f", initial string="at", "Set FIxed F (Oe)") -> (resulting string=w608:string)  [unwired: 1 in, 1 out]
              n140 = call "SetField.vi"("Mode"="Fixed F mode", "Approach"="Fixed Field Approach", "Rate"="FIxed F Rate (Oe/s)", "Field"="Set FIxed F (Oe)", "error in (no error)"=w619, "Instrument Ref In"=w620) -> ("error out"=w615:errorcluster, "Instrument Ref Out"=w617:refnum<k24>)  [unwired: 1 in, 1 out]
              n141 = Divide(x=w597, y=w596) -> (x/y=w595:dbl)
              n142 = local read "F Delay"() -> (w579:dbl)
              n143 = Format Into String(initial string=w609, w603, "Sweep T", w581, w580, w608, w601, w607) -> (resulting string=w611:string)  [unwired: 2 in, 1 out]
              n144 = Multiply(x=w624, y=w595) -> (x*y=w594:dbl)
              n145 = call "WaitFor.vi"("Delay"=w579, "Wait For Field"=TRUE, "error in (no error)"=w615, "Instrument Ref In"=w617) -> ("error out"=w616:errorcluster, "Instrument Ref Out"=w618:refnum<k24>)  [unwired: 6 in]
              n146 = Increment(x=w594) -> (x+1=w593:dbl)
              n147 = String To Path(string=w611) -> (path=w610:path)
              n148 = for {
                N: w593 -> [_]
                tunnel: w625 -> [w645]
                tunnel: w596 -> [w642]
                tunnel: w595 -> [w640]
                tunnel: "Start Value (K)" -> [w643]
                tunnel: "End Value (K)" -> [w641]
                tunnel: w610 -> [w630]
                tunnel: w618 -> [w636]
                tunnel: w616 -> [w635]
                tunnel: w606 -> [w634]
                tunnel: [w633] -> w605
                tunnel: [w632] -> w604
                tunnel: w600 -> [w631]
                tunnel: w589 -> [w629]
                tunnel: w592 -> [w628]
                tunnel: w591 -> [w627]
                tunnel: w590 -> [w626]
                i -> [w639]
                n149 = Less Or Equal?(x=w639, y=w640) -> (x <= y?=w644:bool)
                n150 = case shown="False" w644 {
                  selector: w644 -> [w646 w672]
                  tunnel: w643 -> [w648 w677]
                  tunnel: w639 -> [w657 w676]
                  tunnel: w642 -> [w656 w675]
                  tunnel: [w654 w673] -> w638
                  tunnel: w641 -> [w655 _]
                  tunnel: w640 -> [w650 _]
                  tunnel: w639 -> [w653 _]
                  frame False {
                    n151 = local write "Forward"(w646) -> ()
                    n152 = Not(x=w646) -> (.not. x?=w647:bool)
                    n153 = Multiply(x=w650, y=2) -> (x*y=w649:dbl)
                    n154 = Less Or Equal?(x=w653, y=w649) -> (x <= y?=w651:bool)
                    n155 = local write "Backward"(w647) -> ()
                    n156 = case shown="True" w651 {
                      tunnel: w657 -> [w664 w671]
                      tunnel: w656 -> [w662 w669]
                      tunnel: w655 -> [_ w667]
                      tunnel: [w660 w666] -> w654
                      tunnel: w650 -> [_ w665]
                      tunnel: w649 -> [w659 _]
                      tunnel: w648 -> [w658 _]
                      frame False {
                        n157 = Subtract(x=w664, y=w659) -> (x-y=w663:dbl)
                        n158 = Multiply(x=w662, y=w663) -> (x*y=w661:dbl)
                        n159 = Add(x=w658, y=w661) -> (x+y=w660:dbl)
                      }
                      frame True {
                        n160 = Subtract(x=w671, y=w665) -> (x-y=w670:dbl)
                        n161 = Multiply(x=w669, y=w670) -> (x*y=w668:dbl)
                        n162 = Subtract(x=w667, y=w668) -> (x-y=w666:dbl)
                      }
                    }
                  }
                  frame True {
                    n163 = Multiply(x=w675, y=w676) -> (x*y=w674:dbl)
                    n164 = local write "Forward"(w672) -> ()
                    n165 = Add(x=w677, y=w674) -> (x+y=w673:dbl)
                  }
                }
                n166 = Absolute Value(x=w638) -> (abs(x)=w637:dbl)
                n167 = stacked-sequence {
                  tunnel: w645 -> [_ _ w724]
                  tunnel: w637 -> [w696 _ w720]
                  tunnel: w636 -> [w695 _ _]
                  tunnel: w635 -> [w694 _ _]
                  tunnel: w634 -> [_ w713 w723]
                  tunnel: [w680 _ _] -> w633
                  tunnel: [w679 _ _] -> w632
                  tunnel: w631 -> [_ _ w722]
                  tunnel: w630 -> [_ _ w721]
                  tunnel: w627 -> [_ _ w719]
                  tunnel: w626 -> [_ _ w718]
                  tunnel: w629 -> [_ _ w717]
                  tunnel: w628 -> [_ _ w716]
                  frame #0 {
                    n168 = call "SetTemperature.vi"("Approach"="Sweep Temperature Approach", "Rate"="Sweep T  Rate (K/min)", "Temperature"=w696, "error in (no error)"=w694, "Instrument Ref In"=w695) -> ("error out"=w692:errorcluster, "Instrument Ref Out"=w693:refnum<k24>)  [unwired: 2 in, 1 out]
                    n169 = local read "T Delay"() -> (w678:dbl)
                    n170 = call "WaitFor.vi"("Delay"=w678, "Wait For Temperature"=TRUE ("WaitForTemperature"), "error in (no error)"=w692, "Instrument Ref In"=w693) -> ("error out"=w683:errorcluster, "Instrument Ref Out"=w682:refnum<k24>)  [unwired: 6 in]
                    n171 = for {
                      N: 20 -> [_]
                      shift-right: [w712] -> _
                      shift-left: TRUE -> [w710]
                      shift-right: [w707] -> w680
                      shift-left: w683 -> [w709]
                      tunnel: w682 -> [w706]
                      tunnel: [w704] -> w679
                      tunnel: [w701] -> w689
                      tunnel: [w700] -> w688
                      tunnel: [w702] -> w686 mode=indexing
                      tunnel: [w703] -> w687 mode=indexing
                      n172 = local write "Measuring T"(w710) -> ()
                      n173 = Not(x=w710) -> (.not. x?=w712:bool)
                      n174 = Wait (ms)(milliseconds to wait=u32 200) -> ()  [unwired: 1 out]
                      n175 = call "GetTemperature.vi"("error in (no error)"=w709, "Instrument Ref In"=w706) -> ("Temperature\nStatus"=w700:i32, "Temperature"=w703:dbl, "error out"=w708:errorcluster, "Instrument Ref Out"=w705:refnum<k24>)  [unwired: 3 in, 1 out]
                      n176 = call "GetField.vi"("error in (no error)"=w708, "Instrument Ref In"=w705) -> ("Field\nStatus"=w701:i32, "Field"=w702:dbl, "error out"=w707:errorcluster, "Instrument Ref Out"=w704:refnum<k24>)  [unwired: 3 in, 1 out]
                    }
                    "Field Status" <- w689
                    "Temperature Status" <- w688
                    n177 = call-poly <vilib>:"Mean.vi"("X"=w686) -> ("mean"=→"Fixed Field":dbl)  [unwired: 1 out]
                    n178 = call-poly <vilib>:"Mean.vi"("X"=w687) -> ("mean"=→"Measured Temperature":dbl)  [unwired: 1 out]
                    "Temperature Setting" <- w696
                    "Measuring T" <- FALSE
                  }
                  frame #1 {
                    n179 = Multiply(x=w713, y=1000) -> (x*y=w715:dbl)
                    n180 = Wait (ms)(milliseconds to wait=w715) -> ()  [unwired: 1 out]
                  }
                  frame #2 {
                    n181 = for {
                      N: w717 -> [_]
                      tunnel: w724 -> [w750]
                      tunnel: w720 -> [w746]
                      tunnel: w723 -> [w742]
                      tunnel: w718 -> [w737]
                      tunnel: w719 -> [w735]
                      tunnel: w722 -> [w732]
                      tunnel: w721 -> [w731]
                      tunnel: w720 -> [w730]
                      shift-right: [w749] -> _
                      shift-left: _ -> [w729]
                      shift-right: [w751] -> _
                      shift-left: _ -> [w728]
                      shift-right: [w748] -> _
                      shift-left: _ -> [w727]
                      shift-right: [w726] -> _
                      shift-left: _ -> [w747]
                      tunnel: w716 -> [w725]
                      i -> [w745]
                      n182 = Subtract(x=w735, y=w737) -> (x-y=w739:dbl)
                      n183 = Add(x=0, y=w745) -> (x+y=→"V Loop Run T":i32)
                      n184 = Divide(x=w725, y=1000) -> (x/y=w734:dbl)
                      n185 = Divide(x=w739, y=w734) -> (x/y=w733:dbl)
                      n186 = Multiply(x=2, y=w733) -> (x*y=w738:dbl)
                      n187 = Increment(x=w738) -> (x+1=w736:dbl)
                      n188 = for {
                        N: w736 -> [_]
                        tunnel: w750 -> [w787]
                        tunnel: w746 -> [w782]
                        tunnel: w742 -> [w770]
                        tunnel: w737 -> [w769]
                        tunnel: w735 -> [w768]
                        tunnel: w734 -> [w767]
                        tunnel: w733 -> [w766]
                        tunnel: w732 -> [w764]
                        tunnel: w731 -> [w763]
                        tunnel: w730 -> [w762]
                        shift-right: [w785] -> w749
                        shift-left: w729 -> [w757]
                        shift-right: [w788] -> w751
                        shift-left: w728 -> [w756]
                        shift-right: [w784] -> w748
                        shift-left: w727 -> [w755]
                        shift-right: [w754] -> _
                        shift-left: _ -> [w786]
                        shift-right: [w753] -> w726
                        shift-left: w747 -> [w783]
                        i -> [w765]
                        n189 = flat-sequence {
                          tunnel: w783 -> [w861]
                          tunnel: w786 -> [w862]
                          tunnel: w782 -> [w863]
                          tunnel: w787 -> [w864]
                          tunnel: w756 -> [w865]
                          tunnel: [w865] -> w781
                          tunnel: [w864] -> w779
                          tunnel: [w863] -> w777
                          tunnel: [w862] -> w775
                          tunnel: [w861] -> w773
                          tunnel: [w859] -> w771
                          tunnel: w769 -> [w858]
                          tunnel: w768 -> [w857]
                          tunnel: w767 -> [w856]
                          tunnel: w766 -> [w855]
                          tunnel: w765 -> [w853]
                          tunnel: w781 -> [w904]
                          tunnel: [w904] -> w780
                          tunnel: w779 -> [w897]
                          tunnel: [w896] -> w778
                          tunnel: w777 -> [_]
                          tunnel: [w895] -> w776
                          tunnel: w775 -> [w903]
                          tunnel: [w903] -> w774
                          tunnel: w773 -> [w902]
                          tunnel: [w902] -> w772
                          tunnel: w771 -> [w895]
                          tunnel: [w895] -> w752
                          tunnel: w780 -> [w912]
                          tunnel: [w912] -> w842
                          tunnel: w778 -> [w911]
                          tunnel: [w911] -> w841
                          tunnel: w776 -> [w910]
                          tunnel: [w910] -> w840
                          tunnel: w774 -> [w909]
                          tunnel: [w909] -> w839
                          tunnel: w772 -> [w908]
                          tunnel: [w908] -> w838
                          tunnel: w770 -> [w905]
                          tunnel: [w937] -> w837
                          tunnel: [w924] -> w836
                          tunnel: [w925] -> w835
                          tunnel: [w922] -> w834
                          tunnel: [w925] -> w833
                          tunnel: [w925] -> w832
                          tunnel: [w925] -> w831
                          tunnel: [w925] -> w830
                          tunnel: [w924] -> w829
                          tunnel: [w923] -> w828
                          tunnel: [w922] -> w827
                          tunnel: [w921] -> w826
                          tunnel: ["T Clear Plot B"] -> w825
                          tunnel: ["T Clear Plot A"] -> w824
                          tunnel: [w918] -> w823
                          tunnel: [w917] -> w822
                          tunnel: [w916] -> w821
                          tunnel: [w915] -> w820
                          tunnel: [w914] -> w819
                          tunnel: w842 -> [w913]
                          tunnel: w841 -> [w932]
                          tunnel: w840 -> [w940]
                          tunnel: w839 -> [w939]
                          tunnel: w838 -> [w930]
                          tunnel: w837 -> [w962]
                          tunnel: [w962] -> w818
                          tunnel: w836 -> [w961]
                          tunnel: [w961] -> w817
                          tunnel: w835 -> [w960]
                          tunnel: [w960] -> w816
                          tunnel: w834 -> [w959]
                          tunnel: [w959] -> w815
                          tunnel: w833 -> [w958]
                          tunnel: [w958] -> w814
                          tunnel: w832 -> [w957]
                          tunnel: [w957] -> w813
                          tunnel: w831 -> [w956]
                          tunnel: [w956] -> w812
                          tunnel: w830 -> [w955]
                          tunnel: [w955] -> w811
                          tunnel: w829 -> [w954]
                          tunnel: [w954] -> w810
                          tunnel: w828 -> [w953]
                          tunnel: [w953] -> w809
                          tunnel: w827 -> [w952]
                          tunnel: [w952] -> w808
                          tunnel: w826 -> [w951]
                          tunnel: [w951] -> w807
                          tunnel: w825 -> [w950]
                          tunnel: [w950] -> w806
                          tunnel: w824 -> [w949]
                          tunnel: [w949] -> w805
                          tunnel: w823 -> [w948]
                          tunnel: [w948] -> w804
                          tunnel: w822 -> [w947]
                          tunnel: [w947] -> w803
                          tunnel: w821 -> [w946]
                          tunnel: [w946] -> w802
                          tunnel: w820 -> [w945]
                          tunnel: [w945] -> w801
                          tunnel: w819 -> [w944]
                          tunnel: [w944] -> w800
                          tunnel: w818 -> [w966]
                          tunnel: w817 -> [w1000]
                          tunnel: w816 -> [w999]
                          tunnel: w815 -> [w998]
                          tunnel: w814 -> [w997]
                          tunnel: w813 -> [w995]
                          tunnel: w812 -> [w993]
                          tunnel: w811 -> [w991]
                          tunnel: w810 -> [w988]
                          tunnel: w809 -> [w987]
                          tunnel: w808 -> [w984]
                          tunnel: w807 -> [w983]
                          tunnel: w755 -> [w981]
                          tunnel: w806 -> [w980]
                          tunnel: w757 -> [w978]
                          tunnel: w805 -> [w977]
                          tunnel: w804 -> [w973]
                          tunnel: w803 -> [w972]
                          tunnel: w802 -> [w971]
                          tunnel: w801 -> [w968]
                          tunnel: w800 -> [w967]
                          tunnel: [w966] -> w799
                          tunnel: [w986] -> w798
                          tunnel: [w1000] -> w797
                          tunnel: [w999] -> w796
                          tunnel: [w964] -> w795
                          tunnel: [w965] -> w794
                          tunnel: [w989] -> w793
                          tunnel: [w985] -> w792
                          tunnel: [w982] -> w791
                          tunnel: [w998] -> w790
                          tunnel: [w970] -> w789
                          tunnel: [w1004] -> w758
                          tunnel: [w1005] -> w761
                          tunnel: [w1002] -> w753
                          tunnel: [w1006] -> w784
                          tunnel: [w1007] -> w785
                          tunnel: [w1008] -> _
                          tunnel: [w1009] -> w759
                          tunnel: [w1010] -> w754
                          tunnel: [w1011] -> w760
                          tunnel: [w1001] -> w788
                          tunnel: [w1012] -> _
                          tunnel: w799 -> [w1012]
                          tunnel: w798 -> [w1001]
                          tunnel: w797 -> [w1011]
                          tunnel: w796 -> [w1010]
                          tunnel: w795 -> [w1009]
                          tunnel: w794 -> [w1008]
                          tunnel: w793 -> [w1007]
                          tunnel: w792 -> [w1006]
                          tunnel: w791 -> [w1002]
                          tunnel: w790 -> [w1005]
                          tunnel: w789 -> [w1004]
                          frame #0 {
                            n190 = Less Or Equal?(x=w853, y=w855) -> (x <= y?=w854:bool)
                            n191 = case shown="False" w854 {
                              tunnel: w858 -> [w866 w894]
                              tunnel: w853 -> [w875 w893]
                              tunnel: w856 -> [w874 w892]
                              tunnel: [w872 w890] -> w860
                              tunnel: w857 -> [w873 _]
                              tunnel: w855 -> [w868 _]
                              tunnel: w853 -> [w871 _]
                              frame False {
                                n192 = Multiply(x=w868, y=2) -> (x*y=w867:dbl)
                                n193 = Less Or Equal?(x=w871, y=w867) -> (x <= y?=w869:bool)
                                n194 = case shown="False" w869 {
                                tunnel: w875 -> [w882 w889]
                                tunnel: w874 -> [w880 w887]
                                tunnel: w873 -> [_ w885]
                                tunnel: [w878 w884] -> w872
                                tunnel: w868 -> [_ w883]
                                tunnel: w867 -> [w877 _]
                                tunnel: w866 -> [w876 _]
                                frame False {
                                n195 = Subtract(x=w882, y=w877) -> (x-y=w881:dbl)
                                n196 = Multiply(x=w880, y=w881) -> (x*y=w879:dbl)
                                n197 = Add(x=w876, y=w879) -> (x+y=w878:dbl)
                                }
                                frame True {
                                n198 = Subtract(x=w889, y=w883) -> (x-y=w888:dbl)
                                n199 = Multiply(x=w887, y=w888) -> (x*y=w886:dbl)
                                n200 = Subtract(x=w885, y=w886) -> (x-y=w884:dbl)
                                }
                                }
                              }
                              frame True {
                                n201 = Multiply(x=w892, y=w893) -> (x*y=w891:dbl)
                                n202 = Add(x=w894, y=w891) -> (x+y=w890:dbl)
                              }
                            }
                            n203 = Absolute Value(x=w860) -> (abs(x)=w859:dbl)
                          }
                          frame #1 {
                            n204 = Format Into String(format string="SLVLD1,%.3f;", w895) -> (resulting string=w899:string)  [unwired: 2 in, 1 out]
                            n205 = Concatenate Strings(w899, "\r") -> (w898:string)
                            n206 = VISA Write(VISA resource name=w897, write buffer=w898) -> (VISA resource name out=w896:refnum<visa-resource-name>)  [unwired: 1 in, 2 out]
                            "Sine voltage T" <- w895
                          }
                          frame #2 {
                            n207 = Multiply(x=w905, y=1000) -> (x*y=w907:dbl)
                            n208 = Wait (ms)(milliseconds to wait=w907) -> ()  [unwired: 1 out]
                          }
                          frame #3 {
                            w917 = u8 1 items=["Channel A", "Channel B"] ("Channel A/B for Parameter1")
                            w914 = u8 0 items=["Channel A", "Channel B"] ("Channel A/B for Parameter1")
                            n209 = Format Into String(0) -> (error out=w938:errorcluster)  [unwired: 3 in, 1 out]
                            n210 = Format Into String(0) -> (error out=w933:errorcluster)  [unwired: 3 in, 1 out]
                            n211 = call <instrlib>:"OE1022D_Read 1 parameter_mean.vi"("错误输入（无错误）"=w938, "Parameter"="Parameter A", "Channel (0: A)"=w914, "VISA resource name"=w932) -> ("error out"=w915:errorcluster, "Measurement"=w927:dbl, "VISA resource name out"=w937:refnum<visa-resource-name>)  [unwired: 5 in]
                            n212 = call <instrlib>:"OE1022D_Read 1 parameter_mean.vi"("Parameter 2"="Parameter B", "错误输入（无错误）"=w933, "Channel (0: A)"=w917, "VISA resource name"=w932) -> ("error out"=w918:errorcluster, "Measurement"=w926:dbl, "VISA resource name out"=w916:refnum<visa-resource-name>)  [unwired: 5 in]
                            n213 = Multiply(x=w927, y=1000.0) -> (x*y=w924:dbl)
                            "para1 Measurement (mV)" <- w924
                            n214 = Multiply(x=w926, y=1000000.0) -> (x*y=w922:dbl)
                            "para2 Measurement (uV)" <- w922
                            n215 = Build Array(w924) -> (w941:dbl[])
                            n216 = Build Array(w922) -> (w934:dbl[])
                            n217 = Select(t=w941, s="T Clear Plot A", f=w913) -> (s? t:f=w923:dbl[])
                            n218 = Select(t=w934, s="T Clear Plot B", f=w930) -> (s? t:f=w921:dbl[])
                            n219 = Build Array (concatenate)(w940, w939) -> (w925:dbl[])
                          }
                          frame #4 {
                            n220 = Wait (ms)(milliseconds to wait=u32 50) -> ()  [unwired: 1 out]
                          }
                          frame #5 {
                            n221 = Build Array (concatenate)(w988, w987) -> (w986:dbl[])
                            n222 = Build Array (concatenate)(w984, w983) -> (w982:dbl[])
                            n223 = call <instrlib>:"OE1022D_Read 1 parameter_mean.vi"("错误输入（无错误）"=w968, "Parameter"="Phase A", "Channel (0: A)"=w967, "VISA resource name"=w966) -> ("error out"=w965:errorcluster, "Measurement"=w964:dbl)  [unwired: 5 in, 1 out]
                            "phase A" <- w964
                            n224 = call <instrlib>:"OE1022D_Read 1 parameter_mean.vi"("Parameter 2"="Phase B", "错误输入（无错误）"=w973, "Channel (0: A)"=w972, "VISA resource name"=w971) -> ("Measurement"=w970:dbl)  [unwired: 5 in, 2 out]
                            "phase B" <- w970
                            n225 = Bundle(w993, w986) -> (→"RA-T":cluster{dbl[], dbl[]})  [unwired: 1 in]
                            n226 = Bundle(w995, w982) -> (→"Rh1B-T":cluster{dbl[], dbl[]})  [unwired: 1 in]
                            n227 = Build Array(w964) -> (w974:dbl[])
                            n228 = Build Array(w970) -> (w975:dbl[])
                            n229 = Select(t=w974, s=w977, f=w978) -> (s? t:f=w976:dbl[])
                            n230 = Select(t=w975, s=w980, f=w981) -> (s? t:f=w979:dbl[])
                            n231 = Build Array (concatenate)(w964, w976) -> (w989:dbl[])
                            n232 = Build Array (concatenate)(w970, w979) -> (w985:dbl[])
                            n233 = Bundle(w991, w989) -> (→"PhaseA-T":cluster{dbl[], dbl[]})  [unwired: 1 in]
                            n234 = Bundle(w997, w985) -> (→"Phaseh1-T":cluster{dbl[], dbl[]})  [unwired: 1 in]
                          }
                          frame #6 {
                            n235 = Wait (ms)(milliseconds to wait=u32 50) -> ()  [unwired: 1 out]
                          }
                        }
                        n236 = case shown="True" w764 {
                          tunnel: w763 -> [_ w851]
                          tunnel: w762 -> [_ w848]
                          tunnel: w761 -> [_ w846]
                          tunnel: w760 -> [_ w847]
                          tunnel: w759 -> [_ w845]
                          tunnel: w758 -> [_ w844]
                          tunnel: w752 -> [_ w843]
                          frame False {
                          }
                          frame True {
                            n237 = Build Array(w848, w843, w847, w845, w846, w844) -> (w850:dbl[])
                            n238 = call-poly <vilib>:"Write Delimited Spreadsheet.vi"("file path (dialog if empty)"=w851, "format (%.3f)"="%.10f", "1D data"=w850, "append to file? (new file:F)"=TRUE) -> ()  [unwired: 10 in, 2 out]
                          }
                        }
                      }
                    }
                  }
                }
              }
            }
          }
          "Forward" <- FALSE ("Up")
          "Backward" <- FALSE ("Down")
        }
      }
    }
    frame #2 {
      n239 = case shown="False" "Initialize after measurement" {
        tunnel: w1015 -> [w1016 w1019]
        tunnel: w1014 -> [w1017 w1018]
        frame False {
          n240 = Close Reference(reference=w1017, error in (no error)=w1016) -> ()  [unwired: 1 out]
        }
        frame True {
          w1025 = 0 items=["Linear", "NoOvershoot", "Oscillate"] ("Approach")
          w1026 = 0 items=["Persistent", "Driven"] ("Mode")
          w1022 = 0 items=["FastSettle", "NoOvershoot"] ("Approach")
          n241 = call "SetTemperature.vi"("Approach"=w1022, "Rate"=20.0, "Temperature"=1.6, "error in (no error)"=w1019, "Instrument Ref In"=w1018) -> ("error out"=w1030:errorcluster, "Instrument Ref Out"=w1029:refnum<k24>)  [unwired: 2 in, 1 out]
          n242 = call "SetField.vi"("Mode"=w1026, "Approach"=w1025, "Rate"=200.0, "Field"=0.0, "error in (no error)"=w1030, "Instrument Ref In"=w1029) -> ("error out"=w1027:errorcluster, "Instrument Ref Out"=w1028:refnum<k24>)  [unwired: 1 in, 1 out]
          n243 = Close Reference(reference=w1028, error in (no error)=w1027) -> ()  [unwired: 1 out]
        }
      }
    }
  }
  n244 = while {
    tunnel: w2 -> [w1033]
    tunnel: w1 -> [w1032]
    stop <- "?" stop-if-true
    n245 = for {
      N: 10 -> [_]
      shift-right: [w1048] -> _
      shift-left: w1032 -> [w1050]
      tunnel: w1033 -> [w1047]
      tunnel: [w1045] -> _
      tunnel: [w1042] -> w1039
      tunnel: [w1041] -> w1038
      tunnel: [w1043] -> w1036 mode=indexing
      tunnel: [w1044] -> w1037 mode=indexing
      n246 = call "GetTemperature.vi"("error in (no error)"=w1050, "Instrument Ref In"=w1047) -> ("Temperature\nStatus"=w1041:i32, "Temperature"=w1044:dbl, "error out"=w1049:errorcluster, "Instrument Ref Out"=w1046:refnum<k24>)  [unwired: 3 in, 1 out]
      n247 = Wait (ms)(milliseconds to wait=u32 200) -> ()  [unwired: 1 out]
      n248 = call "GetField.vi"("error in (no error)"=w1049, "Instrument Ref In"=w1046) -> ("Field\nStatus"=w1042:i32, "Field"=w1043:dbl, "error out"=w1048:errorcluster, "Instrument Ref Out"=w1045:refnum<k24>)  [unwired: 3 in, 1 out]
    }
    "Field Status 2" <- w1039
    "Temperature Status 2" <- w1038
    n249 = call-poly <vilib>:"Mean.vi"("X"=w1036) -> ("mean"=→"Field":dbl)  [unwired: 1 out]
    n250 = call-poly <vilib>:"Mean.vi"("X"=w1037) -> ("mean"=→"Temperature":dbl)  [unwired: 1 out]
  }
